vi "niScope Fetch From Digitizing Process.vi"(7 "max wait for packet [ms]":i32=50, 8 "error in":errorcluster, 11 "niScope in":T3={"channel cfg"=[], "sessions"=[], "multi cards"=FALSE, "channels"=0, "type"=enum."n/a", "memory [B/chn]"=0, "ext. clock [Hz]"=0.0, "samples count"=0, "use streaming"=FALSE, "proc setup"={"packet size [smpl]"=0, "current timeout [s]"=0.0, "blk2blk timeout [s]"=0.0, "event time"=timestamp(0 s since 1904-01-01), "temp sampl T [s]"=0.0, "data queue"=refnum, "stop notifier"=refnum, "proc ref"=refnum}, "sample width [B]"=0, "ranges [V]"=[], "trigger setup"={"coupling"=1, "level [V]"=0.0, "slope"=0, "mode"=enum."Immediate"}, "fs [Hz]"=0.0} {"trigger setup"."level [V]" format="%.2f"; "trigger setup"."coupling" items=["AC"=0, "DC"=1, "HF Reject"=3, "LF Reject"=4, "AC Plus HF Reject"=1001]; "channel cfg"."Range [Vpk]" min=0.0; "channel cfg"."Channel" min=0}) -> (0 "error out":errorcluster, 1 "auxiliary sampling data":T1, 2 "data block":T2, 3 "niScope out":T3={"channel cfg"=[], "sessions"=[], "multi cards"=FALSE, "channels"=0, "type"=enum."n/a", "memory [B/chn]"=0, "ext. clock [Hz]"=0.0, "samples count"=0, "use streaming"=FALSE, "proc setup"={"packet size [smpl]"=0, "current timeout [s]"=0.0, "blk2blk timeout [s]"=0.0, "event time"=timestamp(0 s since 1904-01-01), "temp sampl T [s]"=0.0, "data queue"=refnum, "stop notifier"=refnum, "proc ref"=refnum}, "sample width [B]"=0, "ranges [V]"=[], "trigger setup"={"coupling"=1, "level [V]"=0.0, "slope"=0, "mode"=enum."Immediate"}, "fs [Hz]"=0.0} {"trigger setup"."level [V]" format="%.2f"; "trigger setup"."coupling" items=["AC"=0, "DC"=1, "HF Reject"=3, "LF Reject"=4, "AC Plus HF Reject"=1001]; "channel cfg"."Range [Vpk]" min=0.0; "channel cfg"."Channel" min=0}, 4 "fetching done?":bool)   [LabVIEW 2013, in "niScope Virtual Digitizer.lvlib"]
doc: "Tries to fetch data block from digitizing data queue. It waits for predefined amount of time. If fetch timeout is reached it returns no data and no error. If digitizing or fetching timeout is reached it returns timout error. If the last data block was detected it also waits for digitizing process exit. If the process won't return it generates error. If the \ndigitizing process terminates prematurely it will return error. The 'auxiliary sampling data' are valid only if 'valid?' flag in it is True. 'Data block' content is valid only if 'valid?' flag is true. The caller of this VI must collect the data whenever the 'valid?' flag(s) are True. Caller of this VI must always check 'fetching done?' flag and when it is True or function returned error it shall not be called again."
uses:
  niScope Virtual Digitizer.lvlib
  niScope Session.ctl
  niScope Virtual Channel Config.ctl
  niScope Virtual Channel Mode.ctl
  niScope Virtual Channel Input Z.ctl
  niScope Virtual Channel Coupling.ctl
  niScope Type.ctl
  niScope Digitizing Process Options.ctl
  niScope Data Packet.ctl
  niScope Trigger Setup.ctl
  <instrlib>/niScope/Controls/niScope trigger coupling.ctl
  <instrlib>/niScope/Controls/niScope trigger slope.ctl
  niScope Record Aux Data.ctl
  <vilib>/Utility/error.llb/Error Cluster From Error Code.vi
  <vilib>/ErrorRing/Error Ring.xnode
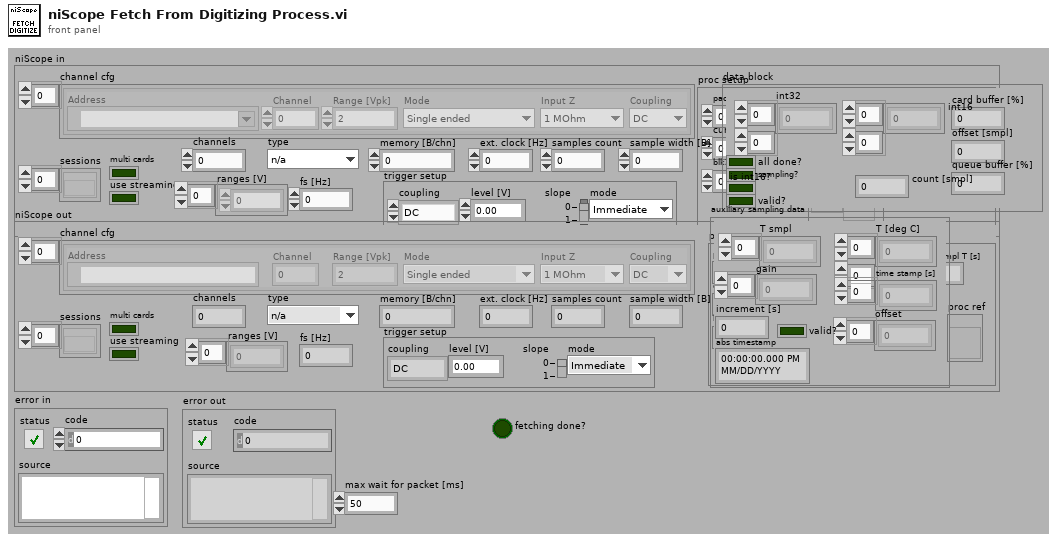
[diagram p1: front panel]
types:
  T1 = typedef "niScope Virtual Digitizer.lvlib/niScope Record Aux Data.ctl" = cluster{"T smpl":i64[], "T [deg C]":dbl[][], "time stamp [s]":dbl[], "offset":dbl[], "gain":dbl[], "increment [s]":dbl, "valid?":bool, "abs timestamp":timestamp}
  T2 = typedef "niScope Virtual Digitizer.lvlib/niScope Data Packet.ctl" = cluster{"int32":i32[][], "card buffer [%]":dbl, "all done?":bool, "offset [smpl]":i64, "sampling?":bool, "queue buffer [%]":dbl, "int16":i16[][], "is int16?":bool, "count [smpl]":i32, "valid?":bool}
  T3 = typedef "niScope Virtual Digitizer.lvlib/niScope Session.ctl" = cluster{"channel cfg":T4[], "sessions":refnum<k20>[], "multi cards":bool, "channels":i32, "type":T8, "memory [B/chn]":i32, "ext. clock [Hz]":dbl, "samples count":i64, "use streaming":bool, "proc setup":T9, "sample width [B]":i32, "ranges [V]":dbl[], "trigger setup":T10, "fs [Hz]":dbl}
  T4 = typedef "niScope Virtual Digitizer.lvlib/niScope Virtual Channel Config.ctl" = cluster{"Address":refnum<k15>, "Channel":i32, "Mode":T5, "Input Z":T6, "Coupling":T7, "Range [Vpk]":dbl}
  T5 = typedef "niScope Virtual Digitizer.lvlib/niScope Virtual Channel Mode.ctl" = enum16{"Single ended", "Unbal. differential", "Differential"}
  T6 = typedef "niScope Virtual Digitizer.lvlib/niScope Virtual Channel Input Z.ctl" = enum16{"1 MOhm", "50 Ohm"}
  T7 = typedef "niScope Virtual Digitizer.lvlib/niScope Virtual Channel Coupling.ctl" = enum16{"AC", "DC", "GND"}
  T8 = typedef "niScope Virtual Digitizer.lvlib/niScope Type.ctl" = enum16{"n/a", "5922"}
  T9 = typedef "niScope Virtual Digitizer.lvlib/niScope Digitizing Process Options.ctl" = cluster{"packet size [smpl]":i64, "current timeout [s]":dbl, "blk2blk timeout [s]":dbl, "event time":timestamp, "temp sampl T [s]":dbl, "data queue":refnum<queue>, "stop notifier":refnum<notifier>, "proc ref":refnum<vi>}
  T10 = typedef "niScope Virtual Digitizer.lvlib/niScope Trigger Setup.ctl" = cluster{"coupling":T11, "level [V]":dbl, "slope":T12, "mode":enum16{"Immediate", "External", "Level"}}
  T11 = typedef "niScope trigger coupling.ctl" = u16
  T12 = typedef "niScope trigger slope.ctl" = i32
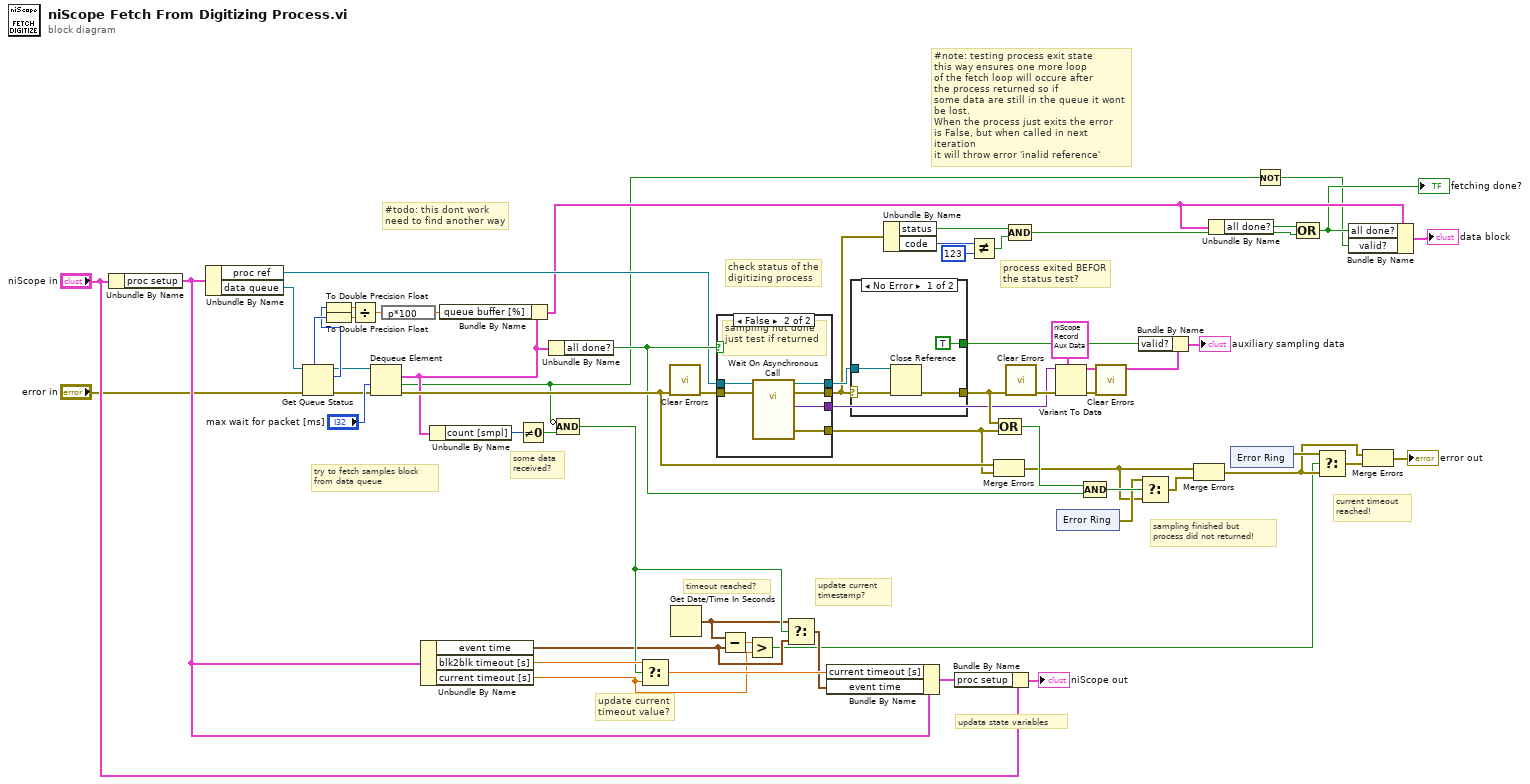
[diagram p0: block diagram]
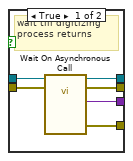
[diagram p3: hidden frame]
diagram:
  # "#note: testing process exit state\nthis way ensures one more loop\nof the fetch loop will occure after\nthe process returned so if\nsome data are still in the queue it wont\nbe lost.\nWhen the process just exits the error\nis False, but when called in next iteration\nit will throw error 'inalid reference'"
  # "process exited BEFOR\nthe status test?"
  # "update current\ntimestamp?"
  # "update current \ntimeout value?"
  # "some data\nreceived?"
  # "#todo: this dont work\nneed to find another way"
  # "updata state variables"
  # "check status of the\ndigitizing process"
  # "try to fetch samples block\nfrom data queue"
  # "current timeout\nreached!"
  # "sampling finished but\nprocess did not returned!"
  # "timeout reached?"
  n1 = Unbundle By Name("niScope in") -> ("proc setup"=w42:T9)
  n2 = Unbundle By Name(w42) -> ("proc ref"=w43:refnum<vi>, "data queue"=w30:refnum<queue>)
  n3 = Get Queue Status(queue=w30, error in (no error)="error in") -> (queue out=w32:refnum<queue>, max queue size=w38:i32, # pending remove=w33:i32, error out=w39:errorcluster)  [unwired: 1 in, 4 out]
  n4 = To Double Precision Float(number=w33) -> (double precision float=w34:dbl)
  n5 = To Double Precision Float(number=w38) -> (double precision float=w35:dbl)
  n6 = Divide(x=w34, y=w35) -> (x/y=w37:dbl)
  n7 = Dequeue Element(queue=w32, timeout in ms (-1)="max wait for packet [ms]", error in (no error)=w39) -> (element=w25:T2, timed out?=w3:bool, error out=w59:errorcluster)  [unwired: 1 out]
  n8 = expression code="p*100"(w37) -> (w36:dbl)
  n9 = Unbundle By Name(w42) -> ("event time"=w19:timestamp, "blk2blk timeout [s]"=w22:dbl, "current timeout [s]"=w1:dbl)
  n10 = Unbundle By Name(w25) -> ("count [smpl]"=w24:i32)
  n11 = Bundle By Name(cluster=w25, "queue buffer [%]"=w36) -> (w27:T2)
  n12 = Not Equal To 0?(x=w24) -> (x != 0?=w23:bool)
  n13 = Unbundle By Name(w25) -> ("all done?"=w50:bool)
  n14 = Compound Arithmetic op=AND(invert w3, w23) -> (w21:bool)
  n15 = Select(t=w22, s=w21, f=w1) -> (s? t:f=w18:dbl)
  n16 = call <vilib>:"Clear Errors.vi"("error in (no error)"=w59) -> ("error out"=w60:errorcluster)  [unwired: 6 in]
  n17 = Get Date/Time In Seconds() -> (seconds since 1Jan1904=w20:timestamp)
  n18 = case shown="False" w50 {
    tunnel: w43 -> [w68 w74]
    tunnel: w60 -> [w67 w73]
    tunnel: [w66 w72] -> w58
    tunnel: [w65 w71] -> w10
    tunnel: [w64 w70] -> w12
    tunnel: [w63 w69] -> w44
    frame True {
      # "wait till digitizing\nprocess returns"
      n19 = call-by-ref "Wait On Asynchronous Call"(reference=w68, error in=w67) -> (reference out=w63:refnum<vi>, error out=w65:errorcluster, 0:"error out"=w66:errorcluster, "auxiliary data out"=w64:variant)  [unwired: 10 in]
    }
    frame False {
      # "sampling not done\njust test if returned"
      n20 = call-by-ref "Wait On Asynchronous Call"(reference=w74, error in=w73) -> (reference out=w69:refnum<vi>, error out=w71:errorcluster, 0:"error out"=w72:errorcluster, "auxiliary data out"=w70:variant)  [unwired: 10 in]
    }
  }
  n21 = Subtract(x=w20, y=w19) -> (x-y=w61:dbl)
  n22 = Greater?(x=w61, y=w1) -> (0:w16:bool)
  n23 = Select(t=w20, s=w21, f=w19) -> (s? t:f=w17:timestamp)
  n24 = Bundle By Name(cluster=w42, "current timeout [s]"=w18, "event time"=w17) -> (w41:T9)
  n25 = case shown="No Error" w10 {
    selector: w10 -> [w78 w79]
    tunnel: [w77 w79] -> w45
    tunnel: w44 -> [w76 _]
    tunnel: [TRUE _] -> w11
    frame No Error {
      n26 = Close Reference(reference=w76, error in (no error)=w78) -> (error out=w77:errorcluster)
    }
    frame Error {
      # "timeout or\nalready eaxited"
    }
  }
  n27 = Unbundle By Name(w10) -> ("status"=w6:bool, "code"=w9:i32)
  n28 = Bundle By Name(cluster="niScope in", "proc setup"=w41) -> (→"niScope out":T3)
  n29 = Not Equal?(x=w9, y=123) -> (x != y?=w7:bool)
  n30 = Merge Errors(w59, w58) -> (w53:errorcluster)
  n31 = Compound Arithmetic op=OR(w45, w58) -> (w56:bool)
  n32 = call <vilib>:"Clear Errors.vi"("error in (no error)"=w45) -> ("error out"=w51:errorcluster)  [unwired: 6 in]
  n33 = Compound Arithmetic op=AND(w6, w7) -> (w5:bool)
  n34 = Variant To Data(error in=w51, type=T1 {"T smpl"=[], "T [deg C]"=[], "time stamp [s]"=[], "offset"=[], "gain"=[], "increment [s]"=0.0, "valid?"=FALSE, "abs timestamp"=timestamp(0 s since 1904-01-01)} ("aux data"), Variant=w12) -> (data=w14:T1, error out=w13:errorcluster)
  n35 = xnode "Error Ring"() -> ("error out"=w54:errorcluster)
  n36 = Compound Arithmetic op=AND(w56, w50) -> (w55:bool)
  n37 = call <vilib>:"Clear Errors.vi"("error in (no error)"=w13) -> ()  [unwired: 6 in, 1 out]
  n38 = Bundle By Name(cluster=w14, "valid?"=w11) -> (→"auxiliary sampling data":T1)
  n39 = Select(t=w54, s=w55, f=w53) -> (s? t:f=w52:errorcluster)
  n40 = Merge Errors(w53, w52) -> (w47:errorcluster)
  n41 = Unbundle By Name(w27) -> ("all done?"=w26:bool)
  n42 = xnode "Error Ring"() -> ("error out"=w49:errorcluster)
  n43 = Not(x=w3) -> (.not. x?=w2:bool)
  n44 = Compound Arithmetic op=OR(w26, w5) -> (w4:bool)
  "fetching done?" <- w4
  n45 = Select(t=w49, s=w16, f=w47) -> (s? t:f=w48:errorcluster)
  n46 = Bundle By Name(cluster=w27, "all done?"=w4, "valid?"=w2) -> (→"data block":T2)
  n47 = Merge Errors(w47, w48) -> (→"error out":errorcluster)
